vi "Set_Vsg1.vi"(7 "Numeric":dbl) -> (3 "Numeric 2":dbl)   [LabVIEW 2013]
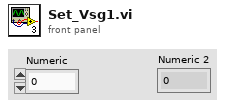
[diagram p1: front panel]
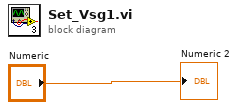
[diagram p0: block diagram]
diagram:
  "Numeric 2" <- "Numeric"
